vi "Write Path to AFG_.exe.vi"(8 "error in (no error)":errorcluster, 10 "Path to AFG*.exe":path, 11 "Wavepond in":refnum<class "Wavepond.lvclass">) -> (0 "error out":errorcluster, 3 "Wavepond out":refnum<class "Wavepond.lvclass">)   [LabVIEW 2014, in "Wavepond.lvclass"]
uses:
  Wavepond.lvclass
  Wavepond.lvclass/Wavepond.ctl
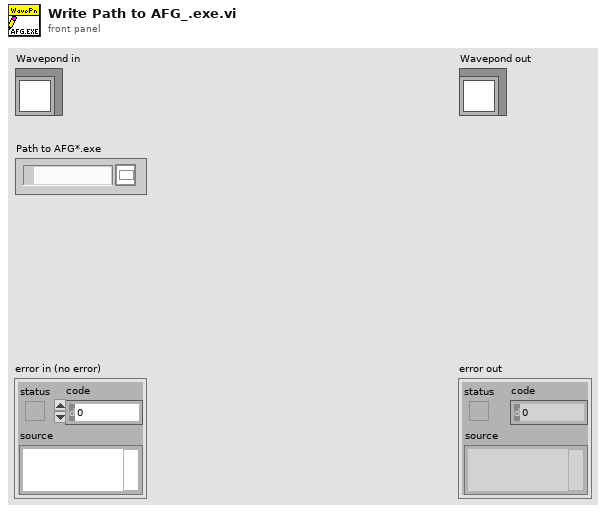
[diagram p1: front panel]
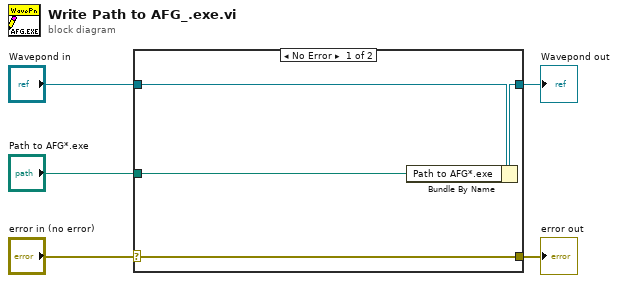
[diagram p0: block diagram]
diagram:
  n1 = case shown="No Error" "error in (no error)" {
    selector: "error in (no error)" -> [w9 w10]
    tunnel: [w9 w10] -> w4
    tunnel: [w7 w11] -> w2
    tunnel: "Wavepond in" -> [w8 w11]
    tunnel: "Path to AFG*.exe" -> [w6 _]
    frame No Error {
      n2 = Bundle By Name(cluster=w8, "Path to AFG*.exe"=w6) -> (w7:refnum<class "Wavepond.lvclass">)
    }
    frame Error {
    }
  }
  "error out" <- w4
  "Wavepond out" <- w2
